vi "UTIL_GetCalConstants.vi"(11 "Full Config":T2) -> (2 "XL Out":string[][](array[string]), 3 "Cal Constants":T1)   [LabVIEW 2024]
uses:
  Control Definitions/Def FullCfg.ctl
  Control Definitions/Def BenchCfg.ctl
  Control Definitions/Def PumpCtlRefs.ctl
  Control Definitions/Def_PumpSpeed.ctl
  Control Definitions/Def Bench Status.ctl
  Control Definitions/DEF_CalConstants.ctl
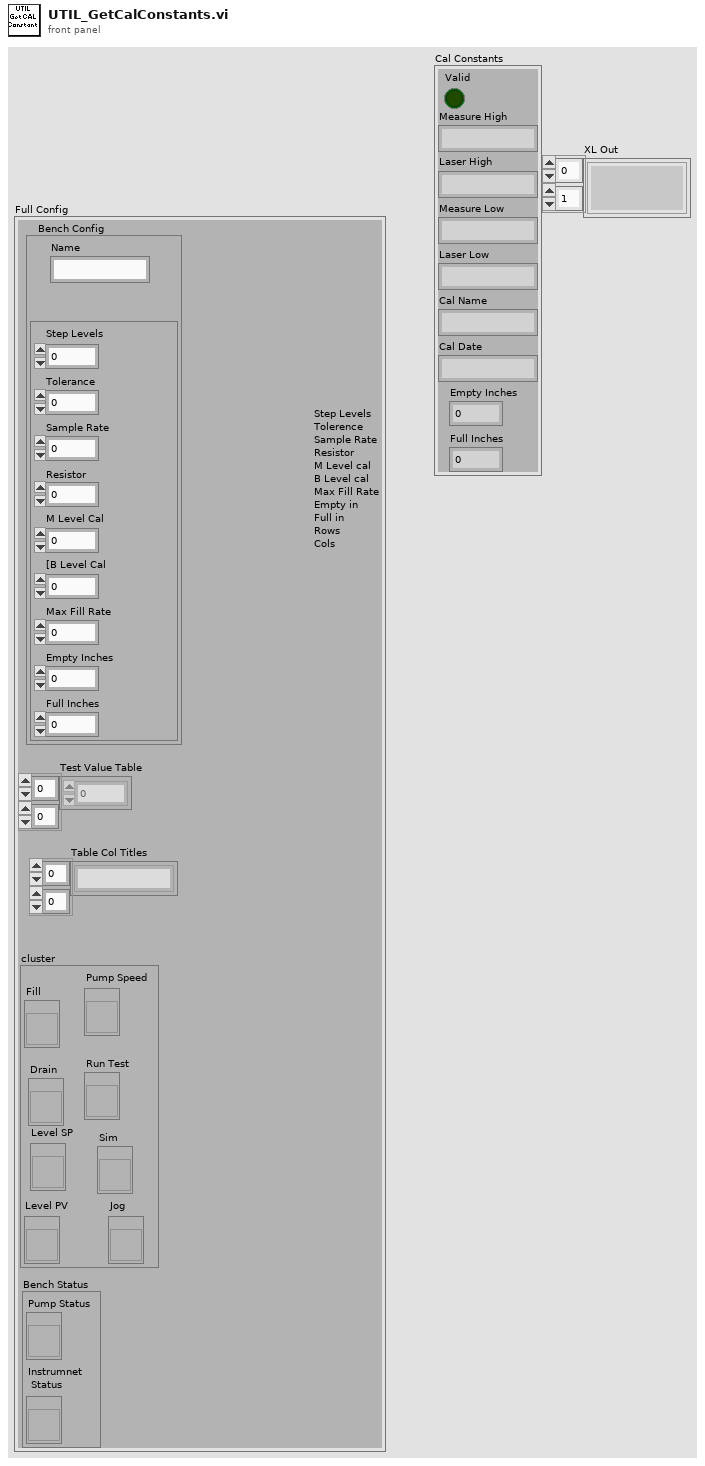
[diagram p1: front panel]
types:
  T1 = typedef "DEF_CalConstants.ctl" = cluster{"Measure High":string, "Laser High":string, "Measure Low":string, "Laser Low":string, "Cal Name":string, "Cal Date":string, "Empty Inches":dbl, "Full Inches":dbl, "Valid":bool}
  T2 = typedef "Def FullCfg.ctl" = cluster{"Bench Config":T3, "Test Value Table ":dbl[][], "Table Col Titles":string[][], "cluster":T4, "Bench Status":T5}
  T3 = typedef "Def BenchCfg.ctl" = cluster{"Name":string, cluster{"Step Levels":dbl, "Tolerance":dbl, "Sample Rate":dbl, "Resistor":dbl, "M Level Cal":dbl, "[B Level Cal":dbl, "Max Fill Rate":dbl, "Empty Inches":dbl, "Full Inches":dbl}}
  T4 = typedef "Def PumpCtlRefs.ctl" = cluster{"Fill ":refnum<vi>, "Drain":refnum<vi>, "Level PV":refnum<vi>, "Pump Speed":refnum<vi>, "Run Test":refnum<vi>, "Sim":refnum<vi>, "Jog":refnum<vi>, "Level SP":refnum<vi>}
  T5 = typedef "Def Bench Status.ctl" = cluster{"Pump Status":refnum<vi>, "Instrumnet\n Status":refnum<vi>}
  T6 = cluster{"Step Levels":dbl, "Tolerance":dbl, "Sample Rate":dbl, "Resistor":dbl, "M Level Cal":dbl, "[B Level Cal":dbl, "Max Fill Rate":dbl, "Empty Inches":dbl, "Full Inches":dbl}
  T7 = cluster{"Value Read":string, "Value Read":string, "Value Read":string, "Value Read":string, "Value Read":string, "Value Read":string, "Empty Inches":dbl, "Full Inches":dbl, "f":bool}
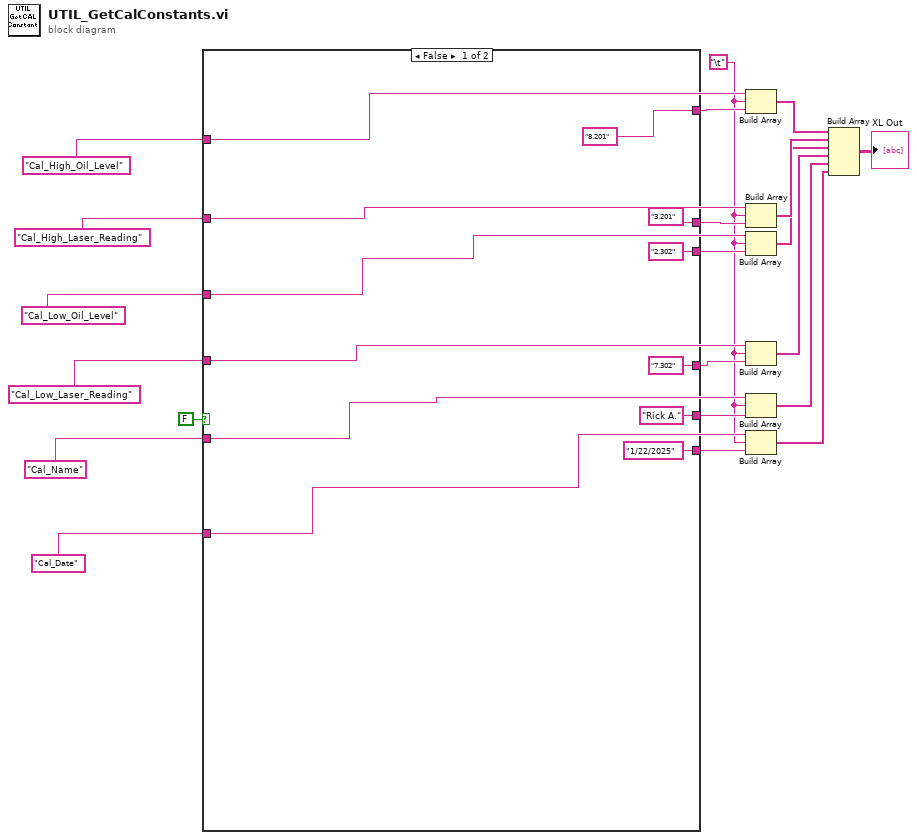
[diagram p0: block diagram]
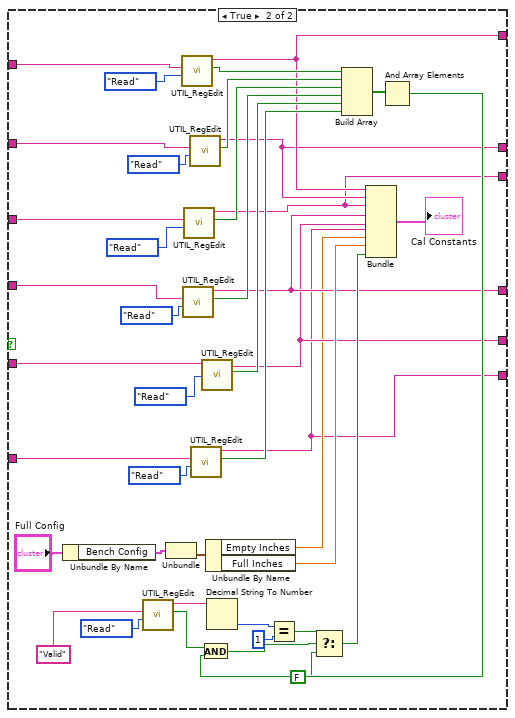
[diagram p2: hidden frame]
diagram:
  w1 = "\t"
  w14 = "Cal_Name"
  w13 = "Cal_Date"
  w21 = "Cal_High_Oil_Level"
  w19 = "Cal_High_Laser_Reading"
  w16 = "Cal_Low_Oil_Level"
  w15 = "Cal_Low_Laser_Reading"
  n1 = case shown="False" FALSE {
    tunnel: w21 -> [_ w40]
    tunnel: ["8.201" ("Value Read") w39] -> w7
    tunnel: w19 -> [_ w38]
    tunnel: ["3.201" ("Value Read") w37] -> w6
    tunnel: w16 -> [_ w36]
    tunnel: ["2.302" ("Value Read") w35] -> w5
    tunnel: w15 -> [_ w34]
    tunnel: ["7.302" ("Value Read") w33] -> w4
    tunnel: w14 -> [_ w32]
    tunnel: ["Rick A." ("Value Read") w31] -> w3
    tunnel: w13 -> [_ w30]
    tunnel: ["1/22/2025" ("Value Read") w28] -> w2
    frame False {
    }
    frame True {
      n2 = Unbundle By Name("Full Config") -> ("Bench Config"=w62:T3)
      n3 = call "UTIL_RegEdit.vi"("Mode"=enum16{"Write", "Read", "Delete"}."Read", "String Name"="Valid") -> ("Success?"=w50:bool, "Value Read"=w48:string)  [unwired: 8 in]
      n4 = Unbundle(w62) -> (w63:T6)  [unwired: 1 out]
      n5 = call "UTIL_RegEdit.vi"("Mode"=enum16{"Write", "Read", "Delete"}."Read", "String Name"=w40) -> ("Success?"=w57:bool, "Value Read"=w39:string)  [unwired: 8 in]
      n6 = call "UTIL_RegEdit.vi"("Mode"=enum16{"Write", "Read", "Delete"}."Read", "String Name"=w34) -> ("Success?"=w54:bool, "Value Read"=w33:string)  [unwired: 8 in]
      n7 = call "UTIL_RegEdit.vi"("Mode"=enum16{"Write", "Read", "Delete"}."Read", "String Name"=w36) -> ("Success?"=w55:bool, "Value Read"=w35:string)  [unwired: 8 in]
      n8 = call "UTIL_RegEdit.vi"("Mode"=enum16{"Write", "Read", "Delete"}."Read", "String Name"=w38) -> ("Success?"=w56:bool, "Value Read"=w37:string)  [unwired: 8 in]
      n9 = call "UTIL_RegEdit.vi"("Mode"=enum16{"Write", "Read", "Delete"}."Read", "String Name"=w30) -> ("Success?"=w52:bool, "Value Read"=w28:string)  [unwired: 8 in]
      n10 = call "UTIL_RegEdit.vi"("Mode"=enum16{"Write", "Read", "Delete"}."Read", "String Name"=w32) -> ("Success?"=w53:bool, "Value Read"=w31:string)  [unwired: 8 in]
      n11 = Unbundle By Name(w63) -> ("Empty Inches"=w29:dbl, "Full Inches"=w60:dbl)
      n12 = Decimal String To Number(string=w48) -> (number=w41:i32)  [unwired: 2 in, 1 out]
      n13 = Equal?(x=w41, y=1) -> (x = y?=w46:bool)
      n14 = Build Array(w57, w56, w55, w54, w53, w52) -> (w51:bool[])
      n15 = And Array Elements(Boolean array=w51) -> (logical AND=w49:bool)
      n16 = And(x=w50, y=w49) -> (x .and. y?=w44:bool)
      n17 = Select(t=w46, s=w44, f=FALSE) -> (s? t:f=w43:bool)
      n18 = Bundle("Value Read"=w39, "Value Read"=w37, "Value Read"=w35, "Value Read"=w33, "Value Read"=w31, "Value Read"=w28, "Empty Inches"=w29, "Full Inches"=w60, "f"=w43) -> (→"Cal Constants":T7)  [unwired: 1 in]
    }
  }
  n19 = Build Array(w21, w1, w7) -> (w20:string[])
  n20 = Build Array(w19, w1, w6) -> (w18:string[])
  n21 = Build Array(w16, w1, w5) -> (w12:string[])
  n22 = Build Array(w15, w1, w4) -> (w11:string[])
  n23 = Build Array(w14, w1, w3) -> (w10:string[])
  n24 = Build Array(w13, w1, w2) -> (w9:string[])
  n25 = Build Array(w20, w18, w12, w11, w10, w9) -> (→"XL Out":string[][])
